vi "test-coord-axis-perf-optimize.vi"() -> ()   [LabVIEW 2019]
uses:
  <vilib>/Rock Robotics/WPI/ThirdParty/JAS_Junk/TrajLib/Trajectory_Library.lvlib
panel:
  out "Run Time":dbl
  # "18.732"
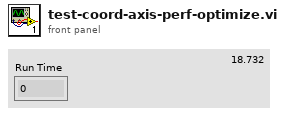
[diagram p1: front panel]
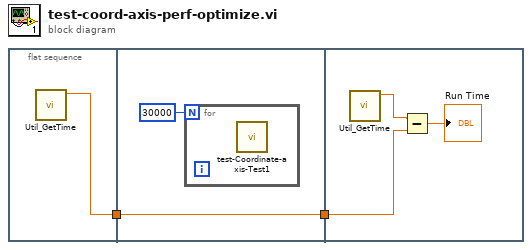
[diagram p0: block diagram]
diagram:
  n1 = flat-sequence {
    tunnel: [w3] -> w1
    tunnel: [w5] -> w2
    tunnel: w1 -> [w5]
    tunnel: w2 -> [w7]
    frame #0 {
      n2 = call <vilib>:"Util_GetTime.vi"() -> ("FPGA_Time_Seconds"=w3:dbl)  [unwired: 10 in, 1 out]
    }
    frame #1 {
      n3 = for {
        N: 30000 -> [_]
        n4 = call "test-Coordinate-axis-Test1.vi"() -> ()  [unwired: 11 in, 1 out]
      }
    }
    frame #2 {
      n5 = call <vilib>:"Util_GetTime.vi"() -> ("FPGA_Time_Seconds"=w8:dbl)  [unwired: 10 in, 1 out]
      n6 = Subtract(x=w8, y=w7) -> (x-y=→"Run Time":dbl)
    }
  }
